vi "Tektronix AFG 1000 Series Generate Standard Waveform.vi"() -> ()   [LabVIEW 2016]
doc: "Demonstrates how to generate a standard waveform."
uses:
  Tektronix AFG 1000 Series.lvlib
panel:
  in  "Phase (0)":dbl
  in  "Duty Cycle (50%)":dbl=50.0
  in  "Channel (1 Channel 1)":u16(ring)=1 items=["Channel 1"=1, "Channel 2"=2]
  in  "Enable Output (T: Enable)":bool=TRUE
  in  "Amplitude (1 Vpp)":dbl=1.0
  in  "DC Offset (0.00 V)":dbl
  in  "Frequency (1000 Hz)":dbl=1000.0
  in  "Waveform Function (0: Sine)":u16(ring) items=["Sine", "Square", "Pulse", "Ramp", "Noise"]
  in  "VISA resource name":refnum<visa-resource-name>
  # "(c) 2016 National Instruments.  ALL RIGHTS RESERVED."
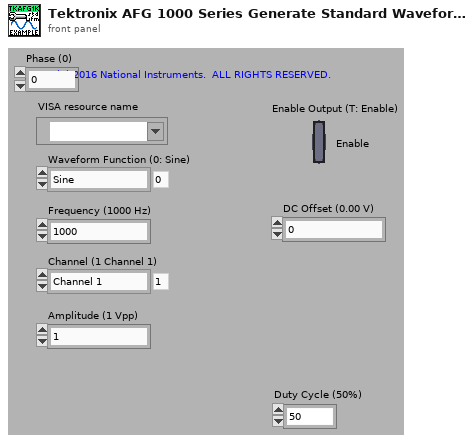
[diagram p1: front panel]
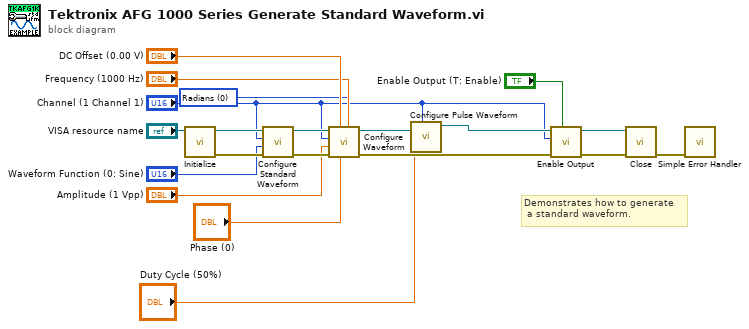
[diagram p0: block diagram]
diagram:
  w5 = u16 0 items=["Radians", "Degrees"] ("Phase Unit (0: Radian)")
  # "Demonstrates how to generate\n a standard waveform."
  n1 = call "Initialize.vi"("VISA resource name"="VISA resource name") -> ("error out"=w19:errorcluster, "VISA resource name out"=w20:refnum<visa-resource-name>)  [unwired: 9 in]
  n2 = call "Configure Standard Waveform.vi"("error in (no error)"=w19, "Waveform Function (0: Sine)"="Waveform Function (0: Sine)", "Channel (1 Channel 1)"="Channel (1 Channel 1)", "VISA resource name"=w20) -> ("error out"=w13:errorcluster, "VISA resource name out"=w11:refnum<visa-resource-name>)  [unwired: 6 in]
  n3 = call "Configure Waveform.vi"("Phase Unit (0: Radian)"=w5, "Frequency (1000 Hz)"="Frequency (1000 Hz)", "Phase (0)"="Phase (0)", "DC Offset (0.00 V)"="DC Offset (0.00 V)", "error in (no error)"=w13, "Amplitude (1 Vpp)"="Amplitude (1 Vpp)", "Channel (1 Channel 1)"="Channel (1 Channel 1)", "VISA resource name"=w11) -> ("error out"=w12:errorcluster, "VISA resource name out"=w4:refnum<visa-resource-name>)  [unwired: 2 in]
  n4 = call "Configure Pulse Waveform.vi"("Duty Cycle (50%)"="Duty Cycle (50%)", "Channel (1: Channel 1)"="Channel (1 Channel 1)", "VISA resource name"=w4) -> ("VISA resource name out"=w3:refnum<visa-resource-name>)  [unwired: 7 in, 1 out]
  n5 = call "Enable Output.vi"("Enable Output (T: Enable)"="Enable Output (T: Enable)", "error in (no error)"=w12, "Channel (1: Channel 1)"="Channel (1 Channel 1)", "VISA resource name"=w3) -> ("error out"=w16:errorcluster, "VISA resource name out"=w17:refnum<visa-resource-name>)  [unwired: 6 in]
  n6 = call "Close.vi"("error in (no error)"=w16, "VISA resource name"=w17) -> ("error out"=w18:errorcluster)  [unwired: 9 in]
  n7 = call <vilib>:"Simple Error Handler.vi"("error in (no error)"=w18) -> ()  [unwired: 4 in, 5 out]
